vi "FTP_Get_Files+Directory_Listing.vi"() -> ()   [LabVIEW 2014]
uses:
  <vilib>/FTP/NI_FTP.lvlib
panel:
  out "Copy Latency":u32
  in  "RT":i32(listbox)
  in  "Stop Button":bool
  in  "Copy Button":bool
  in  "HOST":i32(listbox)
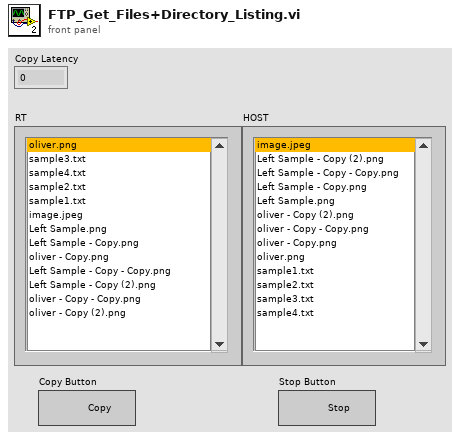
[diagram p1: front panel]
types:
  T1 = typedef "NI_FTP.lvlib/FTP Session.ctl" = refnum<k5>
  T2 = typedef "NI_FTP.lvlib/FTP File Info.ctl" = cluster{"type":enum16{"unknown", "file", "dir", "link"}, "permissions":string, "owner":string, "group":string, "size":i32, "date":string, "name":string, "link name":string}
  T3 = cluster{"remote path":string, "local path":path, "binary":bool}[]
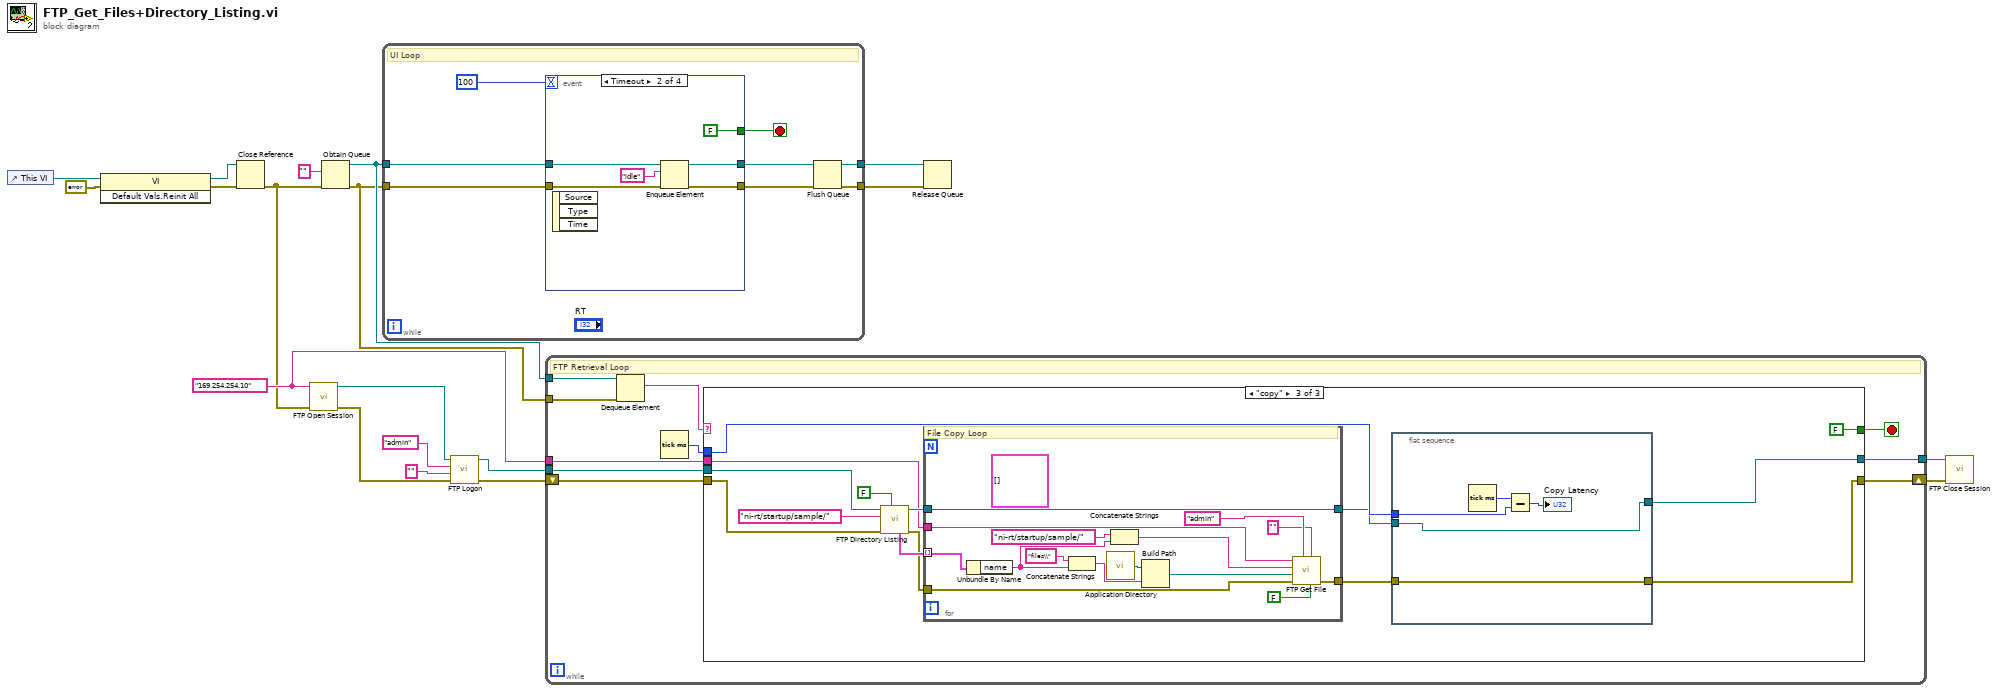
[diagram p0: block diagram]
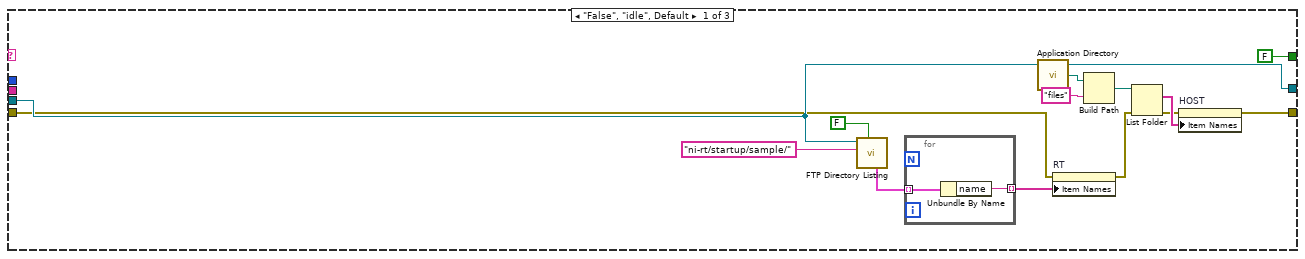
[diagram p2: hidden frame]
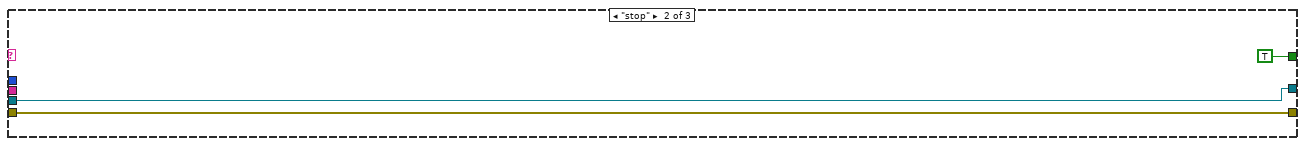
[diagram p3: hidden frame]
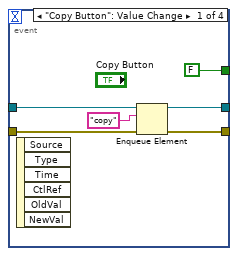
[diagram p4: hidden frame]
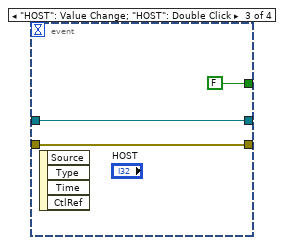
[diagram p5: hidden frame]
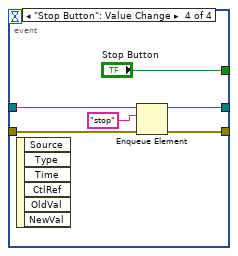
[diagram p6: hidden frame]
diagram:
  w10 = "169.254.254.10" ("address")
  n1 = control-ref of="This VI"() -> (w5:refnum<vi>)
  n2 = invoke class="VI" method="Default Vals.Reinit All"(reference=w5, error in=errorcluster {"status"=FALSE, "code"=0, "source"=""} ("error in (no error)")) -> (reference out=w4:refnum<vi>, error out=w3:errorcluster)  [unwired: 1 in, 1 out]
  n3 = Close Reference(reference=w4, error in (no error)=w3) -> (error out=w1:errorcluster)
  n4 = call <vilib>:"FTP Open Session.vi"("error in (no error)"=w1, "address"=w10) -> ("error out"=w16:errorcluster, "ftp session"=w15:T1)  [unwired: 6 in, 2 out]
  n5 = Obtain Queue(element data type="", error in (no error)=w1) -> (queue out=w7:refnum<queue>, error out=w6:errorcluster)  [unwired: 3 in, 1 out]
  n6 = while {
    tunnel: w7 -> [w27]
    tunnel: w6 -> [w26]
    tunnel: [w23] -> w18
    tunnel: [w22] -> w17
    stop <- w21 stop-if-true
    # "UI Loop"
    n7 = event shown="[1] Timeout" {
      selector: _ -> [_ _ _ _]
      dyn-events: _ -> [_ _ _ _]
      timeout: 100 -> [_ _ _ _]
      tunnel: w27 -> [w33 w37 w41 w47]
      tunnel: w26 -> [w32 w35 w42 w45]
      tunnel: [w30 w38 w41 w46] -> w25
      tunnel: [w29 w39 w42 w44] -> w24
      tunnel: [FALSE ("Stop Button") FALSE ("Stop Button") FALSE ("Stop Button") "Stop Button"] -> w21
      event "Copy Button": Value Change {
        n8 = event-data() -> ()  [unwired: 1 in, 6 out]
        n9 = Enqueue Element(queue=w33, element="copy", error in (no error)=w32) -> (queue out=w30:refnum<queue>, error out=w29:errorcluster)  [unwired: 1 in, 1 out]
      }
      event Timeout {
        n10 = event-data() -> ()  [unwired: 1 in, 3 out]
        n11 = Enqueue Element(queue=w37, element="idle", error in (no error)=w35) -> (queue out=w38:refnum<queue>, error out=w39:errorcluster)  [unwired: 1 in, 1 out]
      }
      event "HOST": Value Change; "HOST": Double Click {
        n12 = event-data() -> ()  [unwired: 1 in, 4 out]
      }
      event "Stop Button": Value Change {
        n13 = event-data() -> ()  [unwired: 1 in, 6 out]
        n14 = Enqueue Element(queue=w47, element="stop", error in (no error)=w45) -> (queue out=w46:refnum<queue>, error out=w44:errorcluster)  [unwired: 1 in, 1 out]
      }
    }
    n15 = Flush Queue(queue=w25, error in (no error)=w24) -> (queue out=w23:refnum<queue>, error out=w22:errorcluster)  [unwired: 1 out]
  }
  n16 = call <vilib>:"FTP Logon.vi"("error in (no error)"=w16, "password"="", "user"="admin", "ftp session"=w15) -> ("error out"=w11:errorcluster, "ftp session out"=w12:T1)  [unwired: 4 in, 2 out]
  n17 = while {
    tunnel: w12 -> [w58]
    tunnel: w10 -> [w56]
    tunnel: [w54] -> w8
    tunnel: w7 -> [w53]
    tunnel: w6 -> [w52]
    shift-right: [w55] -> w9
    shift-left: w11 -> [w57]
    stop <- w50 stop-if-true
    # "FTP Retrieval Loop"
    n18 = Dequeue Element(queue=w53, error in (no error)=w52) -> (element=w51:string)  [unwired: 1 in, 3 out]
    n19 = Tick Count (ms)() -> (millisecond timer value=w49:u32)
    n20 = case shown="\"copy\"" w51 {
      tunnel: w58 -> [w63 w77 w89]
      tunnel: w57 -> [w60 w76 w88]
      tunnel: w56 -> [_ _ w83]
      tunnel: [w66 w76 w81] -> w55
      tunnel: [w63 w77 w79] -> w54
      tunnel: [FALSE TRUE FALSE] -> w50
      tunnel: w49 -> [_ _ w80]
      frame "False", "idle", Default {
        n21 = call <vilib>:"FTP Directory Listing.vi"("active (T)"=FALSE, "directory path"="ni-rt/startup/sample/", "ftp session"=w63) -> ("dir list"=w62:T2[])  [unwired: 4 in, 4 out]
        n22 = for {
          tunnel: w62 -> [w74] mode=indexing
          tunnel: [w73] -> w61 mode=indexing
          n23 = Unbundle By Name(w74) -> ("name"=w73:string)
        }
        n24 = call <vilib>:"Application Directory.vi"() -> ("Application Directory"=w71:path)
        n25 = property on="RT" class="LstBox (strict)"(error in=w60, "Item Names"=w61) -> (error out=w59:errorcluster)  [unwired: 1 in, 1 out]
        n26 = Build Path(base path=w71, name or relative path="files") -> (appended path=w69:path)
        n27 = List Folder(path=w69, error in=w59) -> (filenames=w68:string[], error out=w67:errorcluster)  [unwired: 2 in, 2 out]
        n28 = property on="HOST" class="LstBox (strict)"(error in=w67, "Item Names"=w68) -> (error out=w66:errorcluster)  [unwired: 1 in, 1 out]
      }
      frame "stop" {
      }
      frame "copy" {
        n29 = call <vilib>:"FTP Directory Listing.vi"("active (T)"=FALSE, "error in (no error)"=w88, "directory path"="ni-rt/startup/sample/", "ftp session"=w89) -> ("error out"=w86:errorcluster, "ftp session out"=w85:T1, "dir list"=w87:T2[])  [unwired: 3 in, 2 out]
        n30 = for {
          tunnel: w87 -> [w111] mode=indexing
          tunnel: w85 -> [w108]
          tunnel: [w108] -> w78
          tunnel: w86 -> [w107]
          tunnel: [w106] -> w82
          tunnel: w83 -> [w105]
          (unwired) T3 [] ("file specifications")
          # "File Copy Loop"
          n31 = Unbundle By Name(w111) -> ("name"=w97:string)
          n32 = Concatenate Strings("files\\" ("name or relative path"), w97) -> (w98:string)
          n33 = call <vilib>:"Application Directory.vi"() -> ("Application Directory"=w109:path)
          n34 = Concatenate Strings("ni-rt/startup/sample/" ("directory path"), w97) -> (w104:string)
          n35 = Build Path(base path=w109, name or relative path=w98) -> (appended path=w103:path)
          n36 = call <vilib>:"FTP Get File.vi"("active (T)"=FALSE, "password"="", "user"="admin", "error in (no error)"=w107, "local path"=w103, "remote path"=w104, "host"=w105) -> ("error out"=w106:errorcluster)  [unwired: 3 in, 1 out]
        }
        n37 = flat-sequence {
          tunnel: w82 -> [w96]
          tunnel: w80 -> [w95]
          tunnel: w78 -> [w92]
          tunnel: [w96] -> w81
          tunnel: [w92] -> w79
          frame #0 {
            n38 = Tick Count (ms)() -> (millisecond timer value=w94:u32)
            n39 = Subtract(x=w94, y=w95) -> (x-y=→"Copy Latency":u32)
          }
        }
      }
    }
  }
  n40 = Release Queue(queue=w18, error in (no error)=w17) -> ()  [unwired: 1 in, 3 out]
  n41 = call <vilib>:"FTP Close Session.vi"("error in (no error)"=w9, "ftp session"=w8) -> ()  [unwired: 6 in, 4 out]
